vi "DropPolicyFromString.vi"(6 "Context":string, 8 "error in (no error)":errorcluster, 11 "DropPolicyString":string) -> (0 "error out":errorcluster, 3 "DropPolicy":T1)   [LabVIEW 2026, in "Lumberjack.lvlib"]
uses:
  Lumberjack.lvlib
  TypeDefs/DropPolicy.ctl
  <vilib>/Utility/error.llb/Trim Whitespace (string).vi
  <vilib>/Utility/error.llb/Trim Whitespace One-Sided.vi
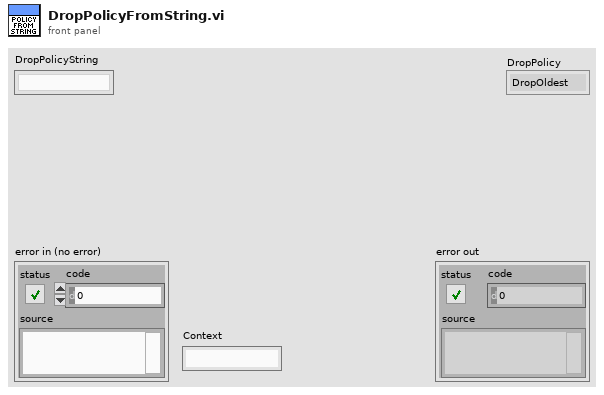
[diagram p1: front panel]
types:
  T1 = typedef "Lumberjack.lvlib/DropPolicy.ctl" = enum16{"DropOldest", "DropNewest", "LevelAware"}
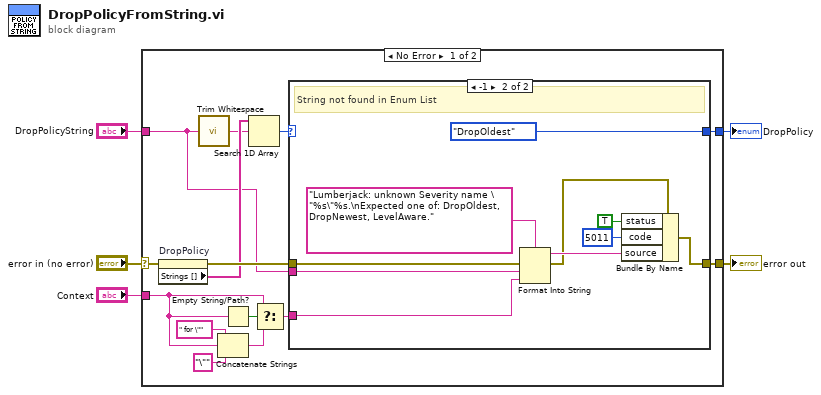
[diagram p0: block diagram]
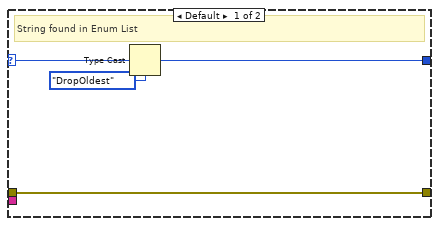
[diagram p2: hidden frame]
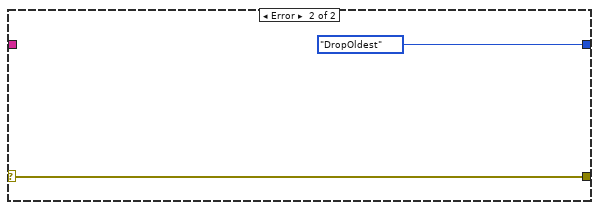
[diagram p3: hidden frame]
diagram:
  n1 = case shown="No Error" "error in (no error)" {
    selector: "error in (no error)" -> [w19 w35]
    tunnel: [w17 w35] -> w5
    tunnel: "DropPolicyString" -> [w7 _]
    tunnel: [w16 DropPolicy."DropOldest" ("DropPolicy")] -> w2
    tunnel: "Context" -> [w9 _]
    frame No Error {
      n2 = property on="DropPolicy" class="Enum (strict)"(error in=w19) -> (error out=w18:errorcluster, "Strings []"=w15:string[])  [unwired: 1 in, 1 out]
      n3 = call-poly <vilib>:"Trim Whitespace.vi"("string"=w7) -> ("trimmed string"=w8:string)  [unwired: 1 in]
      n4 = Concatenate Strings(" for \"" ("string"), w9, "\"" ("string")) -> (w11:string)
      n5 = Empty String/Path?(string/path=w9) -> (empty?=w10:bool)
      n6 = Search 1D Array(1D array=w15, element=w8) -> (index of element=w14:i32)  [unwired: 1 in]
      n7 = Select(t=w9, s=w10, f=w11) -> (s? t:f=w6:string)
      n8 = case shown="-1" w14 {
        selector: w14 -> [w21 _]
        tunnel: w18 -> [w23 w27]
        tunnel: [w23 w26] -> w17
        tunnel: [w22 DropPolicy."DropOldest" ("DropPolicy")] -> w16
        tunnel: w7 -> [_ w25]
        tunnel: w6 -> [_ w24]
        frame Default {
          # "String found in Enum List"
          n9 = Type Cast(type=DropPolicy."DropOldest" ("DropPolicy"), x=w21) -> (*(type *) &x=w22:T1)
        }
        frame -1 {
          # "String not found in Enum List"
          n10 = Format Into String(format string="Lumberjack: unknown Severity name \"%s\"%s.\nExpected one of: DropOldest, DropNewest, LevelAware." ("source"), error in=w27, w25, w24) -> (resulting string=w29:string, error out=w28:errorcluster)  [unwired: 1 in]
          n11 = Bundle By Name(cluster=w28, "status"=TRUE, "code"=5011, "source"=w29) -> (w26:errorcluster)
        }
      }
    }
    frame Error {
    }
  }
  "DropPolicy" <- w2
  "error out" <- w5
